vi "TDC_checkFeatures.vi"(5 "Error In":errorcluster) -> (6 "HiRes":bool, 8 "HBT":bool, 10 "Lifetime":bool, 12 "Channel 0 as 5":bool, 14 "Markers":bool, 15 "Filters":bool, 16 "Ext. Clock":bool, 17 "Dev. Sync.":bool, 18 "Axes":i32, 19 "Error Out":errorcluster)   [LabVIEW 2011]
uses:
  tdcbase.dll
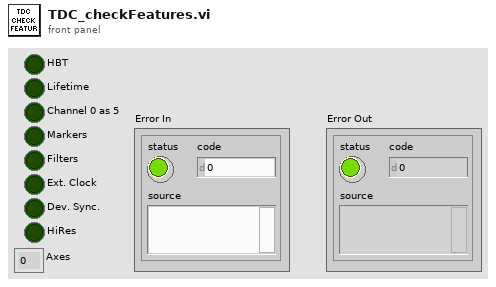
[diagram p1: front panel]
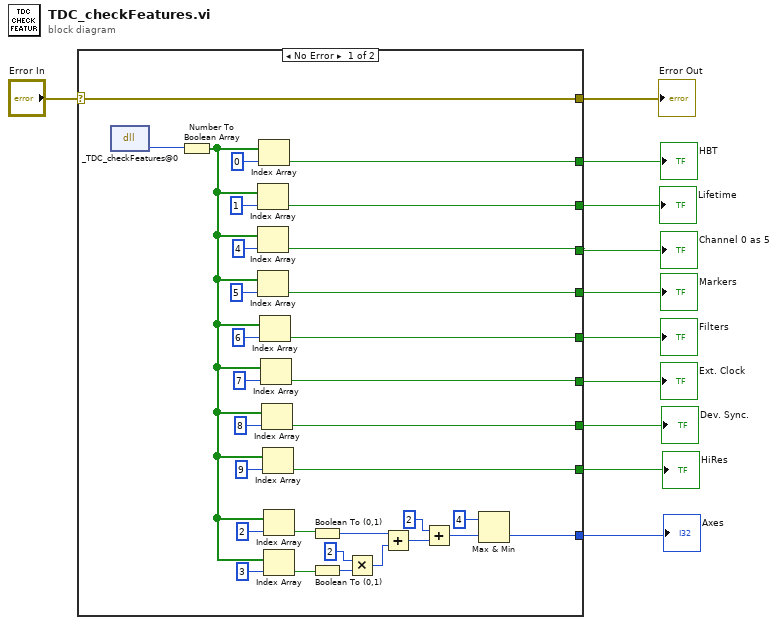
[diagram p0: block diagram]
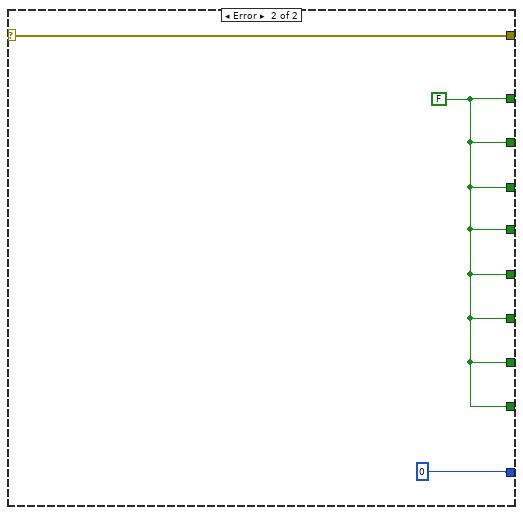
[diagram p2: hidden frame]
diagram:
  n1 = case shown="No Error" "Error In" {
    selector: "Error In" -> [w23 w46]
    tunnel: [w23 w46] -> w10
    tunnel: [w22 0] -> w9
    tunnel: [w21 w44] -> w8
    tunnel: [w20 w44] -> w7
    tunnel: [w19 w44] -> w6
    tunnel: [w18 w44] -> w5
    tunnel: [w17 w44] -> w2
    tunnel: [w16 w44] -> w4
    tunnel: [w15 w44] -> w3
    tunnel: [w12 w44] -> w1
    frame No Error {
      n2 = dll-call lib="X:/tdcbase.dll" fn="_TDC_checkFeatures@0"() -> ("return type"=w24:i32)  [unwired: 3 in, 2 out]
      n3 = Number To Boolean Array(number=w24) -> (Boolean array=w13:bool[])
      n4 = Index Array(array=w13, index=1) -> (element=w16:bool)
      n5 = Index Array(array=w13, index=4) -> (element=w17:bool)
      n6 = Index Array(array=w13, index=5) -> (element=w18:bool)
      n7 = Index Array(array=w13, index=0) -> (element=w15:bool)
      n8 = Index Array(array=w13, index=6) -> (element=w19:bool)
      n9 = Index Array(array=w13, index=7) -> (element=w20:bool)
      n10 = Index Array(array=w13, index=8) -> (element=w21:bool)
      n11 = Index Array(array=w13, index=9) -> (element=w12:bool)
      n12 = Index Array(array=w13, index=2) -> (element=w34:bool)
      n13 = Index Array(array=w13, index=3) -> (element=w35:bool)
      n14 = Boolean To (0,1)(Boolean=w34) -> (0, 1=w39:i16)
      n15 = Boolean To (0,1)(Boolean=w35) -> (0, 1=w36:i16)
      n16 = Multiply(x=2, y=w36) -> (x*y=w38:i32)
      n17 = Add(x=w39, y=w38) -> (x+y=w40:i32)
      n18 = Add(x=2, y=w40) -> (x+y=w42:i32)
      n19 = Max & Min(x=4, y=w42) -> (min(x,y)=w22:i32)  [unwired: 1 out]
    }
    frame Error {
      w44 = FALSE
    }
  }
  "Error Out" <- w10
  "Axes" <- w9
  "HBT" <- w3
  "Lifetime" <- w4
  "Channel 0 as 5" <- w2
  "Markers" <- w5
  "Filters" <- w6
  "Ext. Clock" <- w7
  "Dev. Sync." <- w8
  "HiRes" <- w1
